vi "DataTreeCtrlFM moveData.vi"(5 "movePath":path, 7 "moveNames":string[](array[string]), 8 "error in (no error)":errorcluster, 11 "TDMSAdv Class in":refnum<class "TDMSAdv.lvclass">) -> (0 "error out":errorcluster, 2 "valid":bool, 3 "TDMSAdv Class out":refnum<class "TDMSAdv.lvclass">)   [LabVIEW 2018, in "DataTreeCtrl.lvclass"]
uses:
  DataTreeCtrl.lvclass
  PublicSubVI/Class/FileManager/TDMSAdv.lvclass
  PublicSubVI/Class/FileManager/FM/ctl/_PC_Pub_FM fileReadFuncEnum.ctl
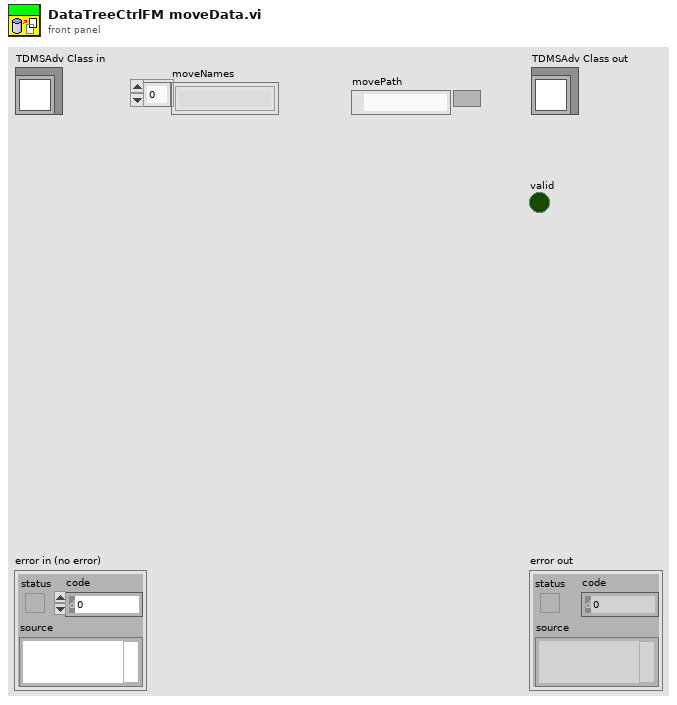
[diagram p1: front panel]
types:
  T1 = typedef "_PC_Pub_FM fileReadFuncEnum.ctl" = enum16{"getAllInfo", "getChromatogram", "getDataItems", "getTimeStamp", "getIdxData", "getIonization", "getRemark", "getAttrFormat"}
  T2 = enum16{"open", "open or create", "create or replace", "create", "open (read-only)"}
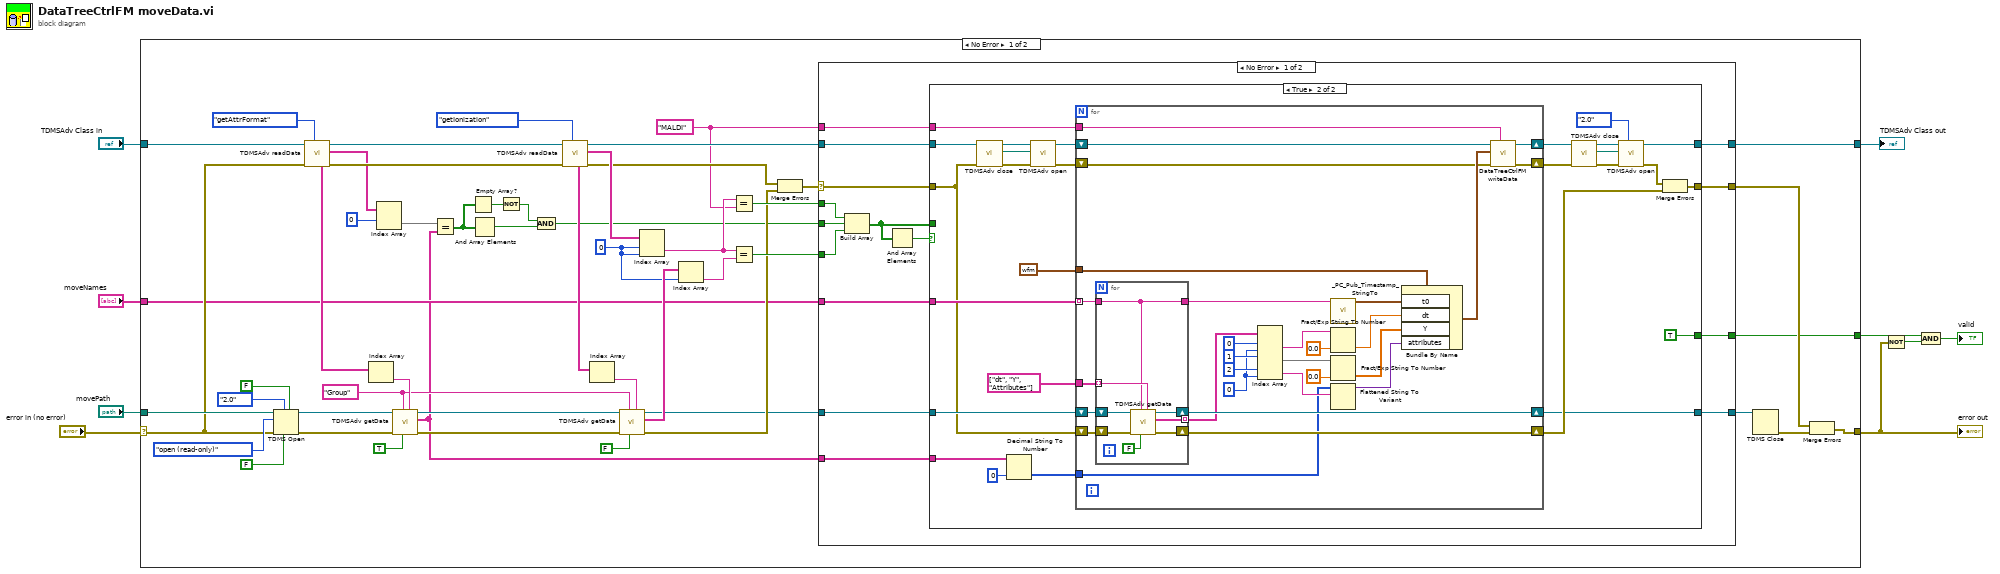
[diagram p0: block diagram]
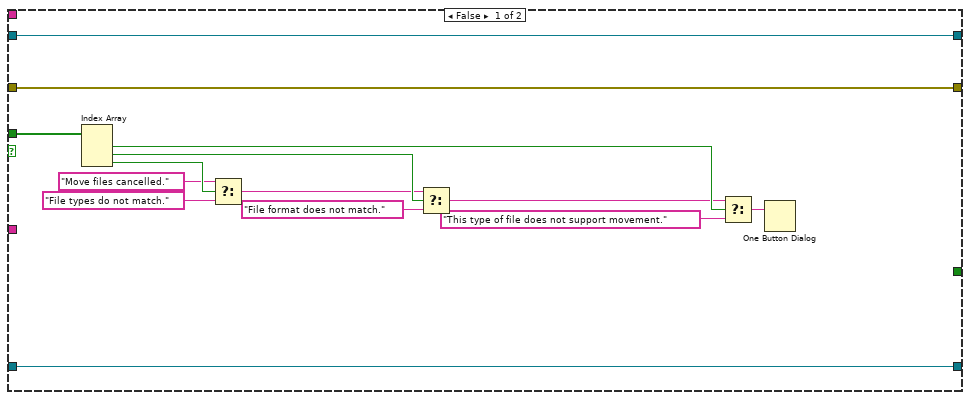
[diagram p2: hidden frame]
diagram:
  n1 = case shown="No Error" "error in (no error)" {
    selector: "error in (no error)" -> [w50 w158]
    tunnel: [w16 w158] -> w4
    tunnel: [w24 w157] -> w7
    tunnel: "TDMSAdv Class in" -> [w51 w157]
    tunnel: "movePath" -> [w56 _]
    tunnel: "moveNames" -> [w23 _]
    tunnel: [w15 _] -> w2
    frame No Error {
      w22 = "MALDI" ("y")
      w34 = 0 ("index (row)")
      w39 = "Group" ("group name")
      n2 = TDMS Open(5:FALSE ("create index file? (T)"), 6:FALSE ("disable buffering (T)"), 7:enum16{"1.0", "2.0"}."2.0" ("file format version (2.0)"), 8:w50, 10:T2."open (read-only)" ("operation"), 11:w56) -> (0:w54:errorcluster, 3:w55:refnum<k34>)  [unwired: 1 in]
      n3 = call "TDMSAdv readData.vi"("readEvent"=_PC_Pub_FM_fileReadFuncEnum."getAttrFormat", "error in (no error)"=w50, "TDMSAdv in"=w51) -> ("error out"=w44:errorcluster, "outputArr"=w38:string[][], "TDMSAdv out"=w45:refnum<class "TDMSAdv.lvclass">, "getListTag"=w43:string[])  [unwired: 5 in]
      n4 = Index Array(array=w43) -> (element=w42:string)  [unwired: 1 in]
      n5 = Index Array(array=w38, index (row)=0) -> (element=w21:string[])  [unwired: 1 in]
      n6 = call "TDMSAdv getData.vi"("channel name"=w42, "stringSplit? (T)"=TRUE, "group name"=w39, "error in (no error)"=w54, "tdms1.0 file"=w55) -> ("error out"=w46:errorcluster, "dataArr"=w20:string[], "tdms1.0 file out"=w47:refnum<k34>)  [unwired: 4 in]
      n7 = Equal?(x=w21, y=w20) -> (x = y?=w14:bool[])
      n8 = Empty Array?(array=w14) -> (empty?=w13:bool)
      n9 = And Array Elements(Boolean array=w14) -> (logical AND=w11:bool)
      n10 = Not(x=w13) -> (.not. x?=w12:bool)
      n11 = And(x=w12, y=w11) -> (x .and. y?=w10:bool)
      n12 = call "TDMSAdv readData.vi"("readEvent"=_PC_Pub_FM_fileReadFuncEnum."getIonization", "error in (no error)"=w44, "TDMSAdv in"=w45) -> ("error out"=w29:errorcluster, "outputArr"=w36:string[][], "TDMSAdv out"=w26:refnum<class "TDMSAdv.lvclass">, "getListTag"=w41:string[])  [unwired: 5 in]
      n13 = Index Array(array=w41) -> (element=w40:string)  [unwired: 1 in]
      n14 = call "TDMSAdv getData.vi"("channel name"=w40, "stringSplit? (T)"=FALSE, "group name"=w39, "error in (no error)"=w46, "tdms1.0 file"=w47) -> ("error out"=w28:errorcluster, "dataArr"=w35:string[], "tdms1.0 file out"=w25:refnum<k34>)  [unwired: 4 in]
      n15 = Index Array(array=w36, index (row)=w34, index (col)=w34) -> (element=w32:string)
      n16 = Index Array(array=w35, index=w34) -> (element=w33:string)
      n17 = Equal?(x=w32, y=w22) -> (x = y?=w31:bool)
      n18 = Equal?(x=w32, y=w33) -> (x = y?=w30:bool)
      n19 = Merge Errors(w29, w28) -> (w27:errorcluster)
      n20 = case shown="No Error" w27 {
        selector: w27 -> [w67 w156]
        tunnel: w31 -> [w75 _]
        tunnel: w10 -> [w74 _]
        tunnel: w30 -> [w73 _]
        tunnel: [w63 w156] -> w17
        tunnel: w26 -> [w70 w155]
        tunnel: w25 -> [w69 w154]
        tunnel: [w68 w155] -> w24
        tunnel: w23 -> [w66 _]
        tunnel: w22 -> [w65 _]
        tunnel: w20 -> [w64 _]
        tunnel: [w62 w154] -> w19
        tunnel: [w61 _] -> w15
        frame No Error {
          n21 = Build Array(w75, w74, w73) -> (w71:bool[])
          n22 = And Array Elements(Boolean array=w71) -> (logical AND=w72:bool)
          n23 = case shown="True" w72 {
            tunnel: w71 -> [w89 _]
            tunnel: w70 -> [w78 w104]
            tunnel: w69 -> [w76 w116]
            tunnel: [w78 w93] -> w68
            tunnel: w67 -> [w77 w103]
            tunnel: w66 -> [_ w115]
            tunnel: w65 -> [_ w114]
            tunnel: w64 -> [_ w113]
            tunnel: [w77 w109] -> w63
            tunnel: [w76 w106] -> w62
            tunnel: [_ TRUE] -> w61
            frame False {
              n24 = Index Array(array=w89) -> (element #1=w88:bool, element #2=w83:bool, element #3=w84:bool)  [unwired: 3 in]
              n25 = Select(t="Move files cancelled.", s=w84, f="File types do not match.") -> (s? t:f=w82:string)
              n26 = Select(t=w82, s=w83, f="File format does not match.") -> (s? t:f=w80:string)
              n27 = Select(t=w80, s=w88, f="This type of file does not support movement.") -> (s? t:f=w79:string)
              n28 = One Button Dialog(message=w79) -> ()  [unwired: 1 in, 1 out]
            }
            frame True {
              n29 = call "TDMSAdv close.vi"("error in (no error)"=w103, "TDMSAdv in"=w104) -> ("error out"=w101:errorcluster, "filePath"=w91:path, "TDMSAdv out"=w102:refnum<class "TDMSAdv.lvclass">)  [unwired: 7 in]
              n30 = Decimal String To Number(string=w113, default (0L)=i16 0 ("default (0 I32)")) -> (number=w112:i16[])  [unwired: 1 in, 1 out]
              n31 = call "TDMSAdv open.vi"("error in (no error)"=w101, "openPath"=w91, "TDMSAdv in"=w102) -> ("error out"=w99:errorcluster, "TDMSAdv out"=w100:refnum<class "TDMSAdv.lvclass">)  [unwired: 7 in]
              n32 = for {
                tunnel: w115 -> [w143] mode=indexing
                shift-right: [w121] -> w96
                shift-left: w100 -> [w122]
                tunnel: string[] ["dt", "Y", "Attributes"] ("getInofList") -> [w142]
                tunnel: w114 -> [w120]
                shift-right: [w141] -> w106
                shift-left: w116 -> [w145]
                shift-right: [w140] -> w107
                shift-left: w103 -> [w144]
                tunnel: w112 -> [w128]
                tunnel: waveform(sgl) {"t0"=timestamp(0 s since 1904-01-01), "dt"=1.0, "Y"=[]} ("signal in") -> [w127]
                shift-right: [w117] -> w95
                shift-left: w99 -> [w118]
                w136 = 0 ("disabled index (col)")
                n33 = for {
                  tunnel: w143 -> [w148]
                  tunnel: w142 -> [w151] mode=indexing
                  shift-right: [w150] -> w141
                  shift-left: w145 -> [w153]
                  shift-right: [w149] -> w140
                  shift-left: w144 -> [w152]
                  tunnel: [w148] -> w134
                  tunnel: [w147] -> w135 mode=indexing
                  n34 = call "TDMSAdv getData.vi"("channel name"=w151, "stringSplit? (T)"=FALSE, "group name"=w148, "error in (no error)"=w152, "tdms1.0 file"=w153) -> ("error out"=w149:errorcluster, "dataArr"=w147:string[], "tdms1.0 file out"=w150:refnum<k34>)  [unwired: 4 in]
                }
                n35 = Index Array(array=w135, index (row) #1=0 ("index (row)"), index (col) #1=w136, index (row) #2=1 ("index (row)"), index (row) #3=2 ("index (row)"), index (col) #3=w136) -> (element #1=w131:string, element #2=w130:string[], element #3=w129:string)  [unwired: 1 in]
                n36 = call "_PC_Pub_Timestamp_StringTo.vi"("Timestring"=w134) -> ("Timestamp"=w123:timestamp)  [unwired: 9 in, 1 out]
                n37 = Fract/Exp String To Number(string=w131, default (0 dbl)=0.0 ("default (0 DBL)")) -> (number=w125:dbl)  [unwired: 2 in, 1 out]
                n38 = Fract/Exp String To Number(string=w130, default (0 dbl)=sgl 0.0 ("default (0 DBL)")) -> (number=w124:sgl[])  [unwired: 2 in, 1 out]
                n39 = Flattened String To Variant(6:w129, 7:w128) -> (3:w126:variant)  [unwired: 1 in, 1 out]
                n40 = Bundle By Name(cluster=w127, "t0"=w123, "dt"=w125, "Y"=w124, "attributes"=w126) -> (w119:waveform(sgl))
                n41 = call "DataTreeCtrlFM writeData.vi"("sampleType"=w120, "error IO"=w118, "SignalData"=w119, "TDMSAdv Class in"=w122) -> ("error out"=w117:errorcluster, "TDMSAdv Class out"=w121:refnum<class "TDMSAdv.lvclass">)  [unwired: 6 in]
              }
              n42 = call "TDMSAdv close.vi"("error in (no error)"=w95, "TDMSAdv in"=w96) -> ("error out"=w97:errorcluster, "filePath"=w90:path, "TDMSAdv out"=w98:refnum<class "TDMSAdv.lvclass">)  [unwired: 7 in]
              n43 = call "TDMSAdv open.vi"("file format version"=enum16{"1.0", "2.0", "Adv"}."2.0", "error in (no error)"=w97, "openPath"=w90, "TDMSAdv in"=w98) -> ("error out"=w94:errorcluster, "TDMSAdv out"=w93:refnum<class "TDMSAdv.lvclass">)  [unwired: 6 in]
              n44 = Merge Errors(w94, w107) -> (w109:errorcluster)
            }
          }
        }
        frame Error {
        }
      }
      n45 = TDMS Close(11:w19) -> (0:w18:errorcluster)  [unwired: 1 in, 1 out]
      n46 = Merge Errors(w17, w18) -> (w16:errorcluster)
    }
    frame Error {
    }
  }
  "error out" <- w4
  "TDMSAdv Class out" <- w7
  n47 = Not(x=w4) -> (.not. x?=w3:bool)
  n48 = And(x=w2, y=w3) -> (x .and. y?=→"valid":bool)
